vi "SelectTrueAddress.vi"(8 "error in (no error)":errorcluster) -> (0 "error out":errorcluster, 3 "元素":string)   [LabVIEW 2014]
uses:
  <vilib>/addons/database/Connection.llb/DB Tools Open Connec (String).vi
  <vilib>/addons/database/Connection.llb/Conn Execute.vi
  <vilib>/addons/database/Recordset.llb/Rec Fetch Recordset Data (R).vi
  <vilib>/addons/database/Recordset.llb/Rec Destroy - Connection.vi
  <vilib>/addons/database/_DB Variant To Data/Database Variant To Data.xnode
  <vilib>/addons/database/NI_Database_API.lvlib
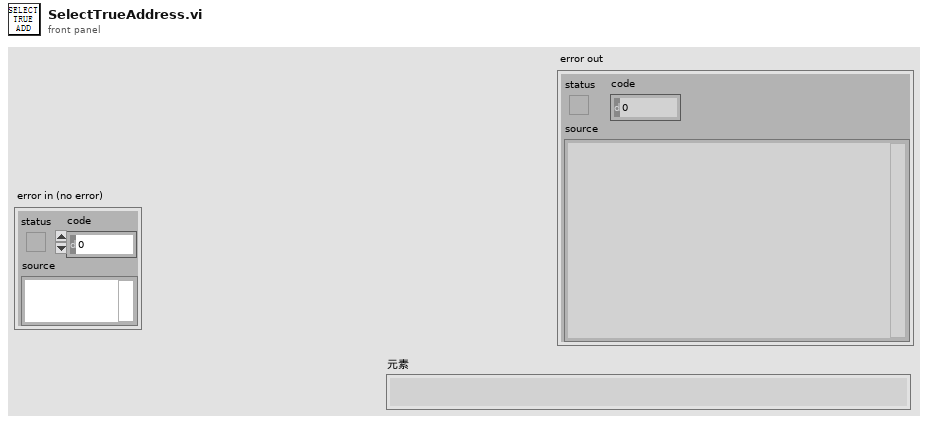
[diagram p1: front panel]
types:
  T1 = typedef "NI_Database_API.lvlib/Conn ObjectReference.ctl" = refnum<k1>
  T2 = typedef "NI_Database_API.lvlib/Rec ObjectReference.ctl" = refnum<k1>
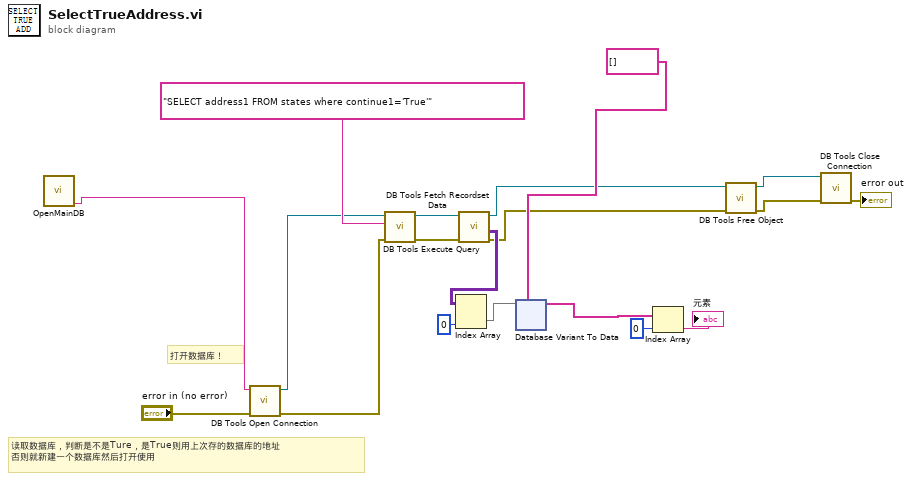
[diagram p0: block diagram]
diagram:
  # "读取数据库，判断是不是Ture，是True则用上次存的数据库的地址\n否则就新建一个数据库然后打开使用"
  # "打开数据库！"
  n1 = call "OpenMainDB.vi"() -> ("头信息"=w1:string)  [unwired: 11 in]
  n2 = call-poly <vilib>:"DB Tools Open Connection.vi"("error in (no error)"="error in (no error)", "connection information"=w1) -> ("error out"=w6:errorcluster, "connection reference"=w5:T1)  [unwired: 6 in]
  n3 = call-poly <vilib>:"DB Tools Execute Query.vi"("error in (no error)"=w6, "SQL query"="SELECT address1 FROM states where continue1='True'", "connection reference"=w5) -> ("error out"=w8:errorcluster, "recordset reference"=w7:T2)  [unwired: 5 in]
  n4 = call-poly <vilib>:"DB Tools Fetch Recordset Data.vi"("error in (no error)"=w8, "recordset reference"=w7) -> ("error out"=w11:errorcluster, "recordset data"=w13:variant[][], "recordset reference out"=w10:T2)  [unwired: 3 in]
  n5 = Index Array(array=w13, index (col)=0 ("index (row)")) -> (element=w14:variant[])  [unwired: 1 in]
  n6 = xnode "Database Variant To Data"("database variant"=w14, "type"=string[] []) -> ("data"=w16:string[])  [unwired: 1 in, 1 out]
  n7 = Index Array(array=w16, index=0 ("索引")) -> (element=→"元素":string)
  n8 = call-poly <vilib>:"DB Tools Free Object.vi"("error in (no error)"=w11, "recordset reference"=w10) -> ("error out"=w3:errorcluster, "connection reference"=w4:T1)  [unwired: 8 in]
  n9 = call <vilib>:"DB Tools Close Connection.vi"("error in (no error)"=w3, "connection reference"=w4) -> ("error out"=→"error out":errorcluster)  [unwired: 5 in]
